vi "Find Personality by Model.vi"(5 "Model":string, 11 "error in (no error)":errorcluster) -> (3 "Version":string, 6 "Personality":u8, 8 "Model ID":u8, 15 "error out":errorcluster)   [LabVIEW 2016]
doc: "This VI searches the config file for the personality defined by model number in the Model Config file."
uses:
  <vilib>/Utility/config.llb/Read Key (String).vi
  <vilib>/Utility/config.llb/Read Key (U32).vi
  <vilib>/Utility/error.llb/Error Cluster From Error Code.vi
  <vilib>/ErrorRing/Error Ring.xnode
  <vilib>/Utility/config.llb/NI_LVConfig.lvlib
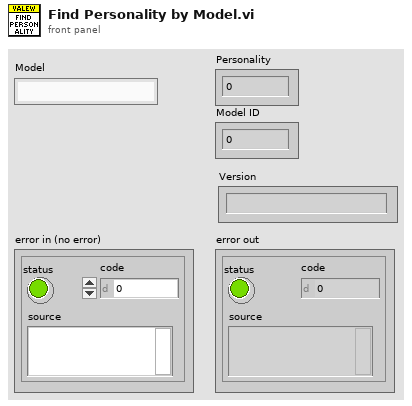
[diagram p1: front panel]
types:
  T1 = typedef "NI_LVConfig.lvlib/Config Data RefNum.ctl" = refnum<k1>
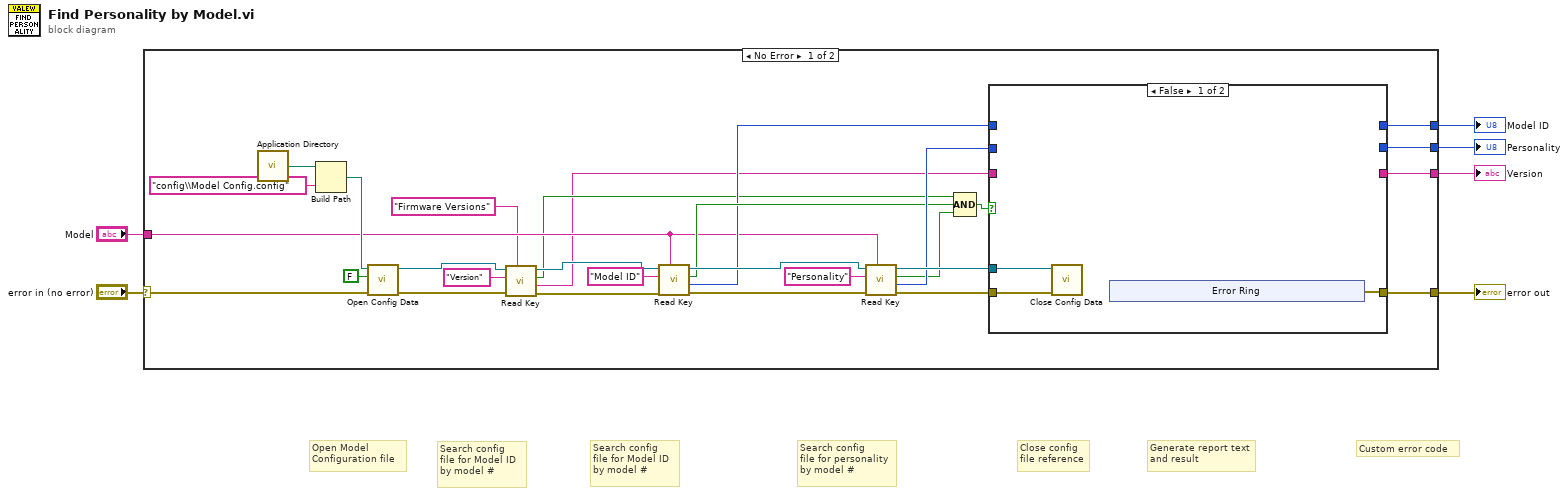
[diagram p0: block diagram]
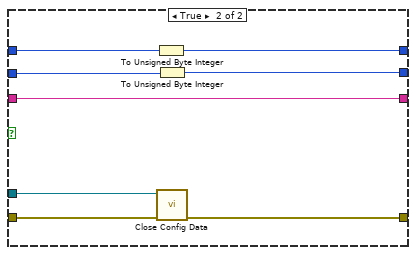
[diagram p2: hidden frame]
diagram:
  # "Search config \nfile for Model ID\nby model #"
  # "Search config \nfile for Model ID\nby model #"
  # "Custom error code"
  # "Generate report text\nand result"
  # "Close config\nfile reference"
  # "Search config \nfile for personality\nby model #"
  # "Open Model \nConfiguration file"
  n1 = case shown="No Error" "error in (no error)" {
    selector: "error in (no error)" -> [w25 w52]
    tunnel: [w34 _] -> w6
    tunnel: [w33 w52] -> w5
    tunnel: "Model" -> [w16 _]
    tunnel: [w17 _] -> w2
    tunnel: [w8 _] -> w1
    frame No Error {
      n2 = call <vilib>:"Application Directory.vi"() -> ("Application Directory"=w29:path)
      n3 = Build Path(base path=w29, name or relative path="config\\Model Config.config") -> (appended path=w28:path)
      n4 = call <vilib>:"Open Config Data.vi"("error in (no error)"=w25, "create file if necessary (T)"=FALSE, "configuration file path"=w28) -> ("error out"=w14:errorcluster, "refnum"=w11:T1)  [unwired: 6 in, 1 out]
      n5 = call-poly <vilib>:"Read Key.vi"("section"="Firmware Versions", "error in (no error)"=w14, "key"="Version", "refnum"=w11) -> ("error out"=w13:errorcluster, "value"=w7:string, "found?"=w9:bool, "refnum out"=w10:T1)  [unwired: 4 in]
      n6 = call-poly <vilib>:"Read Key.vi"("section"=w16, "error in (no error)"=w13, "key"="Model ID", "refnum"=w10) -> ("error out"=w23:errorcluster, "value"=w18:u32, "found?"=w20:bool, "refnum out"=w22:T1)  [unwired: 4 in]
      n7 = call-poly <vilib>:"Read Key.vi"("section"=w16, "error in (no error)"=w23, "key"="Personality", "refnum"=w22) -> ("error out"=w35:errorcluster, "value"=w26:u32, "found?"=w21:bool, "refnum out"=w32:T1)  [unwired: 4 in]
      n8 = Compound Arithmetic op=AND(w9, w20, w21) -> (w19:bool)
      n9 = case shown="False" w19 {
        tunnel: w35 -> [w37 w51]
        tunnel: [_ w50] -> w34
        tunnel: [w38 w49] -> w33
        tunnel: w32 -> [w36 w48]
        tunnel: w26 -> [_ w47]
        tunnel: w18 -> [_ w46]
        tunnel: [_ w45] -> w17
        tunnel: [_ w44] -> w8
        tunnel: w7 -> [_ w44]
        frame False {
          n10 = call <vilib>:"Close Config Data.vi"("error in (no error)"=w37, "refnum"=w36) -> ()  [unwired: 8 in, 2 out]
          n11 = xnode "Error Ring"() -> ("error out"=w38:errorcluster)
        }
        frame True {
          n12 = To Unsigned Byte Integer(number=w46) -> (unsigned 8bit integer=w45:u8)
          n13 = To Unsigned Byte Integer(number=w47) -> (unsigned 8bit integer=w50:u8)
          n14 = call <vilib>:"Close Config Data.vi"("error in (no error)"=w51, "refnum"=w48) -> ("error out"=w49:errorcluster)  [unwired: 8 in, 1 out]
        }
      }
    }
    frame Error {
    }
  }
  "error out" <- w5
  "Personality" <- w6
  "Model ID" <- w2
  "Version" <- w1
